vi "Euler 001.vi"() -> ()   [LabVIEW 2021]
panel:
  out "sum factors 2":i32
  out "sum factors":i32
  in  "root number 2":dbl
  out "sum":i32
  in  "root number":dbl
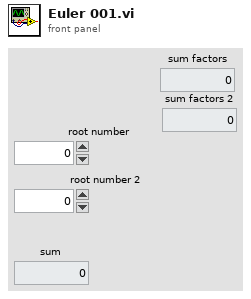
[diagram p1: front panel]
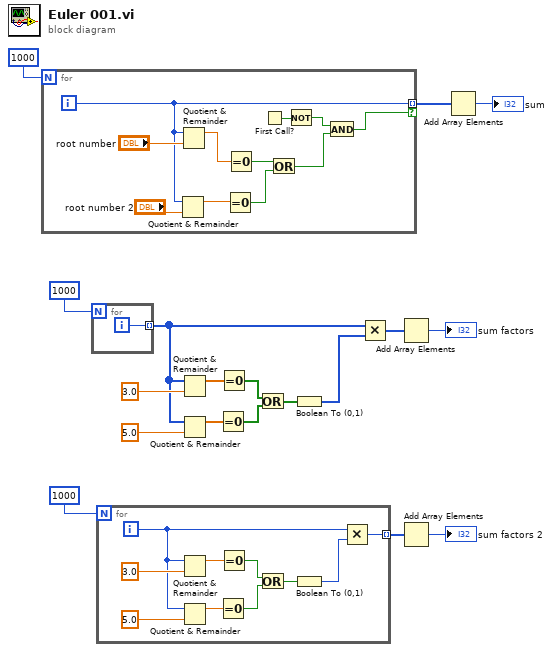
[diagram p0: block diagram]
diagram:
  n1 = for {
    N: 1000 -> [_]
    tunnel: [w22] -> w18 mode=indexing if=w24
    i -> [w22]
    n2 = Quotient & Remainder(x=w22, y="root number 2") -> (x-y*floor(x/y)=w21:dbl)  [unwired: 1 out]
    n3 = Quotient & Remainder(x=w22, y="root number") -> (x-y*floor(x/y)=w28:dbl)  [unwired: 1 out]
    n4 = Equal To 0?(x=w21) -> (x = 0?=w19:bool)
    n5 = Equal To 0?(x=w28) -> (x = 0?=w26:bool)
    n6 = First Call?() -> (First Call?: T/F=w27:bool)
    n7 = Or(x=w26, y=w19) -> (x .or. y?=w20:bool)
    n8 = Not(x=w27) -> (.not. x?=w25:bool)
    n9 = And(x=w25, y=w20) -> (x .and. y?=w24:bool)
  }
  n10 = for {
    N: 1000 -> [_]
    tunnel: [w30] -> w7 mode=indexing
    i -> [w30]
  }
  n11 = for {
    N: 1000 -> [_]
    tunnel: [w40] -> w5 mode=indexing
    i -> [w31]
    n12 = Quotient & Remainder(x=w31, y=3.0 ("root number")) -> (x-y*floor(x/y)=w35:dbl)  [unwired: 1 out]
    n13 = Quotient & Remainder(x=w31, y=5.0 ("root number 4")) -> (x-y*floor(x/y)=w33:dbl)  [unwired: 1 out]
    n14 = Equal To 0?(x=w33) -> (x = 0?=w37:bool)
    n15 = Equal To 0?(x=w35) -> (x = 0?=w36:bool)
    n16 = Or(x=w36, y=w37) -> (x .or. y?=w38:bool)
    n17 = Boolean To (0,1)(Boolean=w38) -> (0, 1=w39:i16)
    n18 = Multiply(x=w31, y=w39) -> (x*y=w40:i32)
  }
  n19 = Quotient & Remainder(x=w7, y=3.0 ("root number")) -> (x-y*floor(x/y)=w14:dbl[])  [unwired: 1 out]
  n20 = Quotient & Remainder(x=w7, y=5.0 ("root number 4")) -> (x-y*floor(x/y)=w16:dbl[])  [unwired: 1 out]
  n21 = Equal To 0?(x=w16) -> (x = 0?=w12:bool[])
  n22 = Equal To 0?(x=w14) -> (x = 0?=w13:bool[])
  n23 = Or(x=w13, y=w12) -> (x .or. y?=w9:bool[])
  n24 = Boolean To (0,1)(Boolean=w9) -> (0, 1=w8:i16[])
  n25 = Multiply(x=w7, y=w8) -> (x*y=w6:i32[])
  n26 = Add Array Elements(numeric array=w6) -> (sum=→"sum factors":i32)
  n27 = Add Array Elements(numeric array=w5) -> (sum=→"sum factors 2":i32)
  n28 = Add Array Elements(numeric array=w18) -> (sum=→"sum":i32)
